vi "initDriver_setTrigger_softwareControl.vi"() -> ()   [LabVIEW 2014]
panel:
  in  "Num Bytes to Fetch (64)":u16=64 min=1
  in  "Address (0x50)":u16=80 max=1023 format="%.0x"
  in  "Aardvark Handle":i32 min=0
  out "error out":errorcluster
  in  "error in (no error)":errorcluster
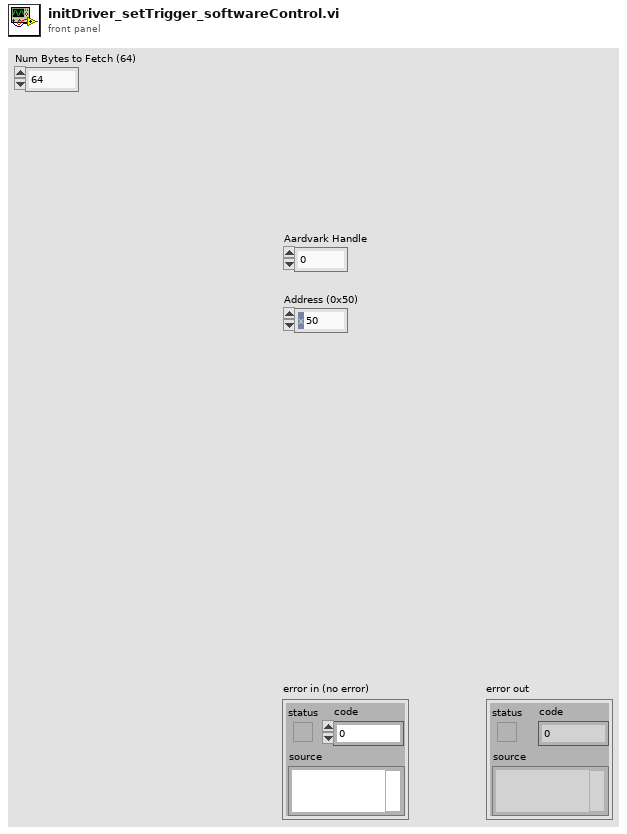
[diagram p1: front panel]
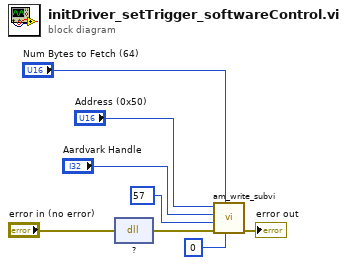
[diagram p0: block diagram]
diagram:
  n1 = dll-call lib="?" fn="?"(error in="error in (no error)") -> (error out=w7:errorcluster)  [unwired: 3 in, 1 out]
  n2 = call "am_write_subvi.vi"("Data to Write"=0, "Num Bytes to Fetch (64)"="Num Bytes to Fetch (64)", "error in (no error)"=w7, "Memory ADD"=u8 57, "Aardvark Handle in"="Aardvark Handle", "Address (0x50) in"="Address (0x50)") -> ("error out"=→"error out":errorcluster)  [unwired: 4 in, 1 out]
